vi "Serial.vi"(8 "error in (no error)":errorcluster, 9 "Clear Log":bool, 10 "write buffer":string="UA[3]\r\n", 11 "VISA resource name":refnum<visa-resource-name>="COM6") -> (0 "error out":errorcluster, 2 "read buffer":string)   [LabVIEW 2017]
uses:
  <vilib>/Instr/_visa.llb/VISA Configure Serial Port (Instr).vi
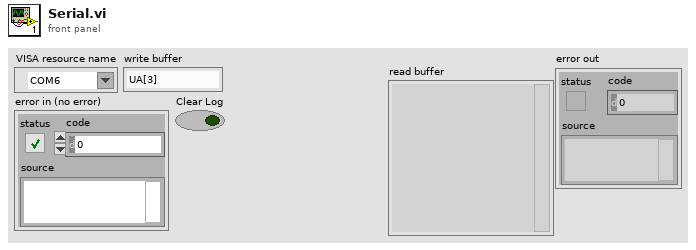
[diagram p1: front panel]
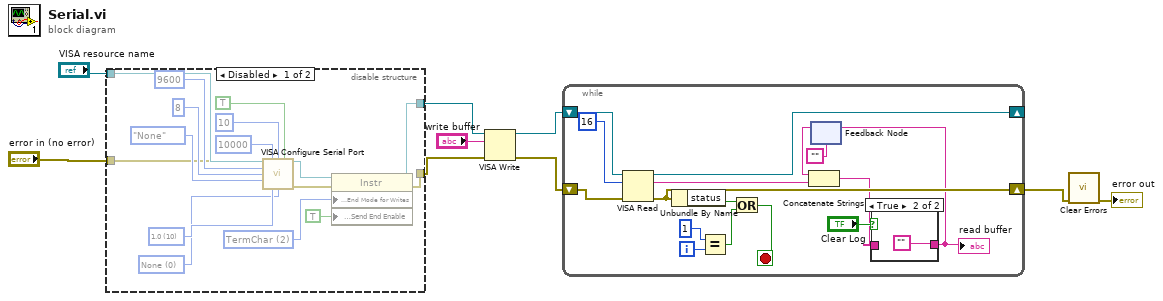
[diagram p0: block diagram]
diagram:
  n1 = disable-structure shown="Disabled" {
    disable-tunnel: "VISA resource name" -> [w25 w27]
    disable-tunnel: "error in (no error)" -> [w19 w26]
    disable-tunnel: [w14 w27] -> w4
    disable-tunnel: [w13 w26] -> w6
    frame Disabled {
      w11 = u16 2 items=["None", "LastBit", "TermChar", "Break"] ("Serial Settings:Serial End Mode for Writes")
      w17 = u16 0 items=["None", "XON/XOFF", "RTS/CTS", "XON/XOFF & RTS/CTS", "DTR/DSR", "XON/XOFF & DTR/DSR"] ("flow control (0:none)")
      w18 = u16 10 items=["1.0"=10, "1.5"=15, "2.0"=20] ("stop bits (10: 1 bit)")
      n2 = call-poly "VISA Configure Serial Port"("VISA resource name"=w25, "timeout (10sec)"=u32 10000, "termination char\n(0xA = '\\n' = LF)"=u8 10 ("termination char\n(0xA = '\\n' = LF)"), "Enable Termination\nChar (T)"=TRUE ("Enable Termination\nChar (T)"), "baud rate (9600)"=u32 9600, "data bits (8)"=u16 8, "parity (0:none)"=enum16{"None", "Odd", "Even", "Mark", "Space"}."None", "error in (no error)"=w19, "stop bits (10: 1 bit)"=w18, "flow control (0:none)"=w17) -> ("VISA resource name out"=w15:refnum<visa-resource-name>, "error out"=w16:errorcluster)  [unwired: 4 in]
      n3 = property class="Instr"(reference=w15, error in=w16, "Serial Settings:End Mode for Writes"=w11, "Message Based Settings:Send End Enable"=TRUE) -> (reference out=w14:refnum<visa-resource-name>, error out=w13:errorcluster)
    }
    frame Enabled {
    }
  }
  n4 = VISA Write(VISA resource name=w4, write buffer="write buffer", error in (no error)=w6) -> (VISA resource name out=w3:refnum<visa-resource-name>, error out=w2:errorcluster)  [unwired: 1 out]
  n5 = while {
    shift-right: [w43] -> _
    shift-left: w3 -> [w34]
    shift-right: [w38] -> w1
    shift-left: w2 -> [w33]
    i -> [w41]
    stop <- w36 stop-if-true
    n6 = VISA Read(VISA resource name=w34, byte count=u32 16, error in (no error)=w33) -> (VISA resource name out=w43:refnum<visa-resource-name>, read buffer=w42:string, error out=w38:errorcluster)  [unwired: 1 out]
    n7 = Unbundle By Name(w38) -> ("status"=w35:bool)
    n8 = Equal?(x=1, y=w41) -> (x = y?=w37:bool)
    n9 = Or(x=w35, y=w37) -> (x .or. y?=w36:bool)
    n10 = feedback #1("") -> (w32:string)
    n11 = Concatenate Strings(w32, w42) -> (w29:string)
    n12 = case shown="True" "Clear Log" {
      tunnel: w29 -> [w44 _]
      tunnel: [w44 ""] -> w28
      frame False {
      }
      frame True {
      }
    }
    "read buffer" <- w28
    n13 = feedback-in #1(w28) -> ()
  }
  n14 = call <vilib>:"Clear Errors.vi"("error in (no error)"=w1) -> ("error out"=→"error out":errorcluster)  [unwired: 5 in, 1 out]
